vi "Close.vi"(8 "error in (no error)":errorcluster, 11 "N5222A PNA in":refnum<class "N5222A PNA.lvclass">) -> (0 "error out":errorcluster, 3 "N5222A PNA out":refnum<class "N5222A PNA.lvclass">)   [LabVIEW 2018, in "N5222A PNA.lvclass"]
uses:
  N5222A PNA.lvclass
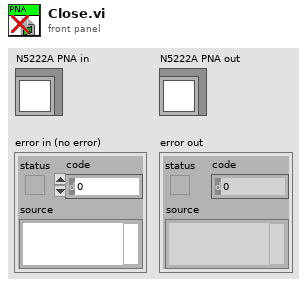
[diagram p1: front panel]
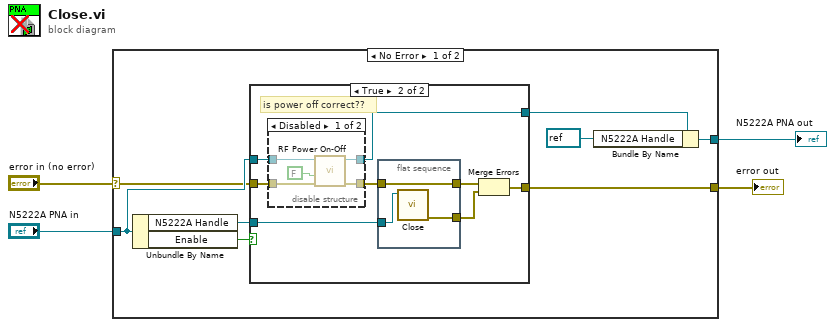
[diagram p0: block diagram]
diagram:
  n1 = case shown="No Error" "error in (no error)" {
    selector: "error in (no error)" -> [w8 w34]
    tunnel: [w7 w34] -> w3
    tunnel: [w10 w33] -> w1
    tunnel: "N5222A PNA in" -> [w9 w33]
    frame No Error {
      n2 = Unbundle By Name(w9) -> ("N5222A Handle"=w12:refnum<visa-resource-name>, "Enable"=w6:bool)
      n3 = case shown="True" w6 {
        tunnel: w12 -> [_ w22]
        tunnel: w9 -> [w13 w21]
        tunnel: w8 -> [w14 w20]
        tunnel: [w14 w18] -> w7
        tunnel: [w13 w15] -> w5
        frame False {
        }
        frame True {
          # "is power off correct??"
          n4 = disable-structure shown="Disabled" {
            disable-tunnel: w21 -> [w27 w29]
            disable-tunnel: w20 -> [w26 w28]
            disable-tunnel: [w25 w28] -> w17
            disable-tunnel: [w24 w29] -> w15
            frame Disabled {
              n5 = call "RF Power On-Off.vi"("error in (no error)"=w26, "RF Power State (T: On)"=FALSE, "N5222A PNA in"=w27) -> ("error out"=w25:errorcluster, "N5222A PNA out"=w24:refnum<class "N5222A PNA.lvclass">)  [unwired: 7 in]
            }
            frame Enabled {
            }
          }
          n6 = flat-sequence {
            tunnel: w22 -> [w32]
            tunnel: [w31] -> w19
            tunnel: [w30] -> w16
            tunnel: w17 -> [w30]
            frame #0 {
              n7 = call <instrlib>:"Close.vi"("VISA Resource Name"=w32) -> ("Error Out"=w31:errorcluster)  [unwired: 10 in]
            }
          }
          n8 = Merge Errors(w16, w19) -> (w18:errorcluster)
        }
      }
      n9 = Bundle By Name(cluster=w5, "N5222A Handle"=refnum<visa-resource-name> refnum) -> (w10:refnum<class "N5222A PNA.lvclass">)
    }
    frame Error {
    }
  }
  "error out" <- w3
  "N5222A PNA out" <- w1
